vi "ReadSF.vi"(0 "connection ID in":refnum<k5>, 1 "enabled":bool, 2 "bytes to read":i32, 3 "header size":i32, 4 "error in":errorcluster) -> (5 "connection ID out":refnum<k5>, 6 "string":string, 7 "error out":errorcluster)   [LabVIEW 2010]
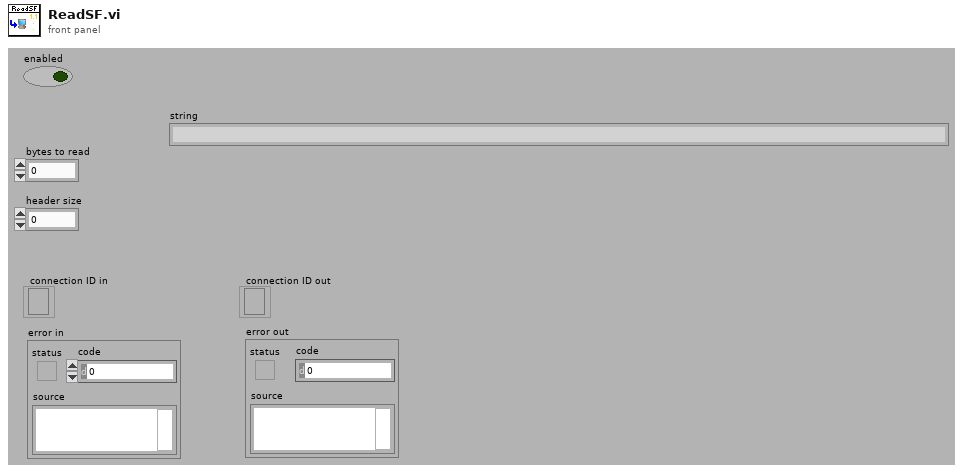
[diagram p1: front panel]
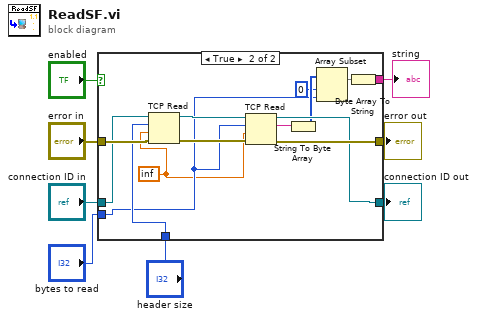
[diagram p0: block diagram]
diagram:
  n1 = case shown="True" "enabled" {
    tunnel: [w10 w24] -> w8
    tunnel: "error in" -> [w10 w18]
    tunnel: "connection ID in" -> [w9 w15]
    tunnel: [w9 w23] -> w4
    tunnel: "bytes to read" -> [_ w12]
    tunnel: "header size" -> [_ w14]
    tunnel: [_ w19] -> w1
    frame False {
    }
    frame True {
      w11 = inf
      n2 = TCP Read(connection ID=w15, bytes to read=w14, error in (no error)=w18, 9:w11) -> (connection ID out=w16:refnum<k5>, error out=w17:errorcluster)  [unwired: 1 in, 1 out]
      n3 = TCP Read(connection ID=w16, bytes to read=w12, error in (no error)=w17, 9:w11) -> (connection ID out=w23:refnum<k5>, data out=w22:string, error out=w24:errorcluster)  [unwired: 1 in]
      n4 = String To Byte Array(string=w22) -> (unsigned byte array=w21:u8[])
      n5 = Array Subset(array=w21, index=0, length=w12) -> (w20:u8[])
      n6 = Byte Array To String(unsigned byte array=w20) -> (string=w19:string)
    }
  }
  "error out" <- w8
  "connection ID out" <- w4
  "string" <- w1
